vi "Mean2D.vi"(1 "Scan":dbl[][](array[numeric]) format="%.2f") -> (0 "mean":dbl format="%.2f")   [LabVIEW 2009]
uses:
  <vilib>/Analysis/NI_AALBase.lvlib
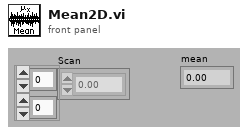
[diagram p1: front panel]
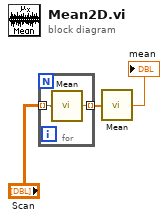
[diagram p0: block diagram]
diagram:
  n1 = for {
    tunnel: "Scan" -> [w5] mode=indexing
    tunnel: [w4] -> w1 mode=indexing
    n2 = call <vilib>:"Mean.vi"("X"=w5) -> ("mean"=w4:dbl)  [unwired: 1 out]
  }
  n3 = call <vilib>:"Mean.vi"("X"=w1) -> ("mean"=→"mean":dbl)  [unwired: 1 out]
